vi "EEPROM Read .vi"(8 "error in (no error)":errorcluster, 10 "client ptr":u32, 11 "Estyx device name":string) -> (0 "error out":errorcluster, 2 "EEPROM data":string[](array[string]))   [LabVIEW 2010, in "lib1299.lvlib"]
doc: "This VI reads the contents of the EEPROM located on the device EVM (daughtercard).\n\nInputs:\nclient ptr - estyx client pointer to file system\nestyx device name - estyx directory name of the device\nTest mode (debug) - allow for testing without EEPROM input. User must supply string to parse.\n\nOutputs:\nRead Data - cluster of information read from the EEPROM\n - Raw Data: contents of eepage 1 date file from estyx\n - Parsed Data: Raw Data parsed based on memory range for the data value (defined on wiki page for EEPROM information)\n - Data - String: EEPROM data derived from finding the string terminator for each of the Parse Data lines"
uses:
  lib1299.lvlib
  Styx/lvstyx/Read/lvstyx_read_all_path.vi
panel:
  # "Name"
  # "PWB"
  # "PCA"
  # "BOM"
  # "Build Date"
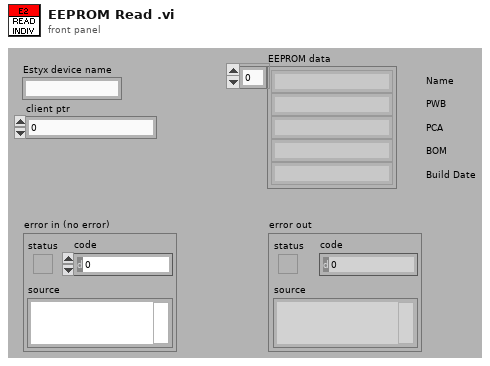
[diagram p1: front panel]
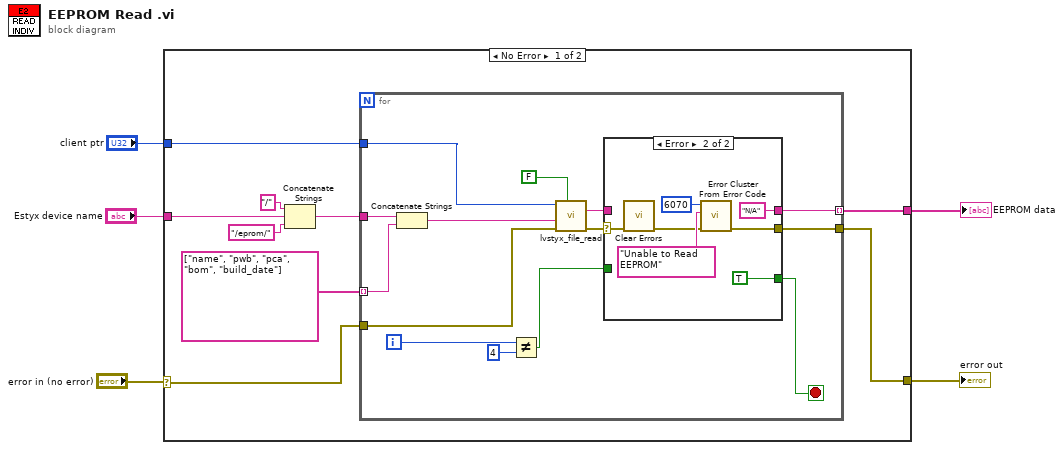
[diagram p0: block diagram]
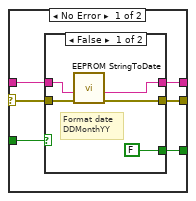
[diagram p2: hidden frame]
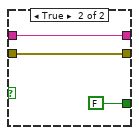
[diagram p3: hidden frame]
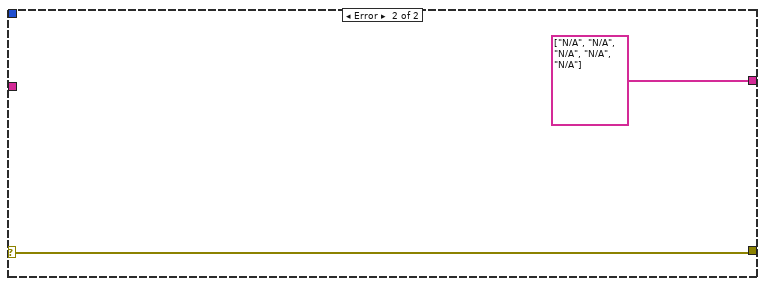
[diagram p4: hidden frame]
diagram:
  n1 = case shown="No Error" "error in (no error)" {
    selector: "error in (no error)" -> [w7 w51]
    tunnel: "Estyx device name" -> [w12 _]
    tunnel: "client ptr" -> [w9 _]
    tunnel: [w8 string[] ["N/A", "N/A", "N/A", "N/A", "N/A"]] -> w3
    tunnel: [w6 w51] -> w1
    frame No Error {
      n2 = Concatenate Strings("/" ("string"), w12, "/eprom/" ("string")) -> (w10:string)
      n3 = for {
        tunnel: string[] ["name", "pwb", "pca", "bom", "build_date"] -> [w27] mode=indexing
        tunnel: w10 -> [w28]
        tunnel: w9 -> [w19]
        tunnel: [w26] -> w8 mode=indexing
        tunnel: w7 -> [w17]
        tunnel: [w20] -> w6
        i -> [w24]
        stop <- w15 stop-if-true
        n4 = Concatenate Strings(w28, w27) -> (w18:string)
        n5 = Not Equal?(x=w24, y=4) -> (x != y?=w25:bool)
        n6 = call-poly "lvstyx_file_read.vi"("Log? (T)"=FALSE ("Notify? (F)"), "error in (no error)"=w17, "path"=w18, "client ptr"=w19) -> ("error out"=w16:errorcluster, "buf"=w22:string)  [unwired: 5 in, 1 out]
        n7 = case shown="Error" w16 {
          selector: w16 -> [w30 w44]
          tunnel: [w34 "N/A" ("buf")] -> w26
          tunnel: w25 -> [w33 _]
          tunnel: w22 -> [w32 _]
          tunnel: [w31 w47] -> w20
          tunnel: [w29 TRUE] -> w15
          frame No Error {
            n8 = case shown="False" w33 {
              tunnel: w32 -> [w39 w42]
              tunnel: [w38 w42] -> w34
              tunnel: w30 -> [w37 w41]
              tunnel: [w36 w41] -> w31
              tunnel: [FALSE FALSE] -> w29
              frame False {
                # "Format date\nDDMonthYY"
                n9 = call "EEPROM StringToDate.vi"("error in (no error)"=w37, "Date String"=w39) -> ("error out"=w36:errorcluster, "Date"=w38:string)  [unwired: 8 in]
              }
              frame True {
              }
            }
          }
          frame Error {
            n10 = call <vilib>:"Clear Errors.vi"("error in (no error)"=w44) -> ("error out"=w43:errorcluster)  [unwired: 6 in]
            n11 = call <vilib>:"Error Cluster From Error Code.vi"("error in (no error)"=w43, "error message (\"\")"="Unable to Read EEPROM" ("error message (\"\")"), "error code (0)"=6070) -> ("error out"=w47:errorcluster)  [unwired: 6 in]
          }
        }
      }
    }
    frame Error {
    }
  }
  "EEPROM data" <- w3
  "error out" <- w1
